vi "test.vi"() -> ()   [LabVIEW 2024]
uses:
  src/Zero Timeout Message Handler/~Message/~Message.lvclass
  PID Loop/PID Loop/PID Loop.lvclass
  PID Loop/PID Loop/Loop Msg/Loop Msg.lvclass
  C:/Users/uspoaotto/OneDrive - Oregon Tool/Desktop/working copies/zeroTimeoutMessageHandler/src/Zero Timeout Message Handler/~Message/~Message.lvclass
  src/Zero Timeout Message Handler/Start Polling Msg/Start Polling Msg.lvclass
  src/Zero Timeout Message Handler/Set Polling Message Msg/Set Polling Message Msg.lvclass
  src/Zero Timeout Message Handler/Stop Polling Msg/Stop Polling Msg.lvclass
  src/Zero Timeout Message Handler/Stop Msg/Stop Msg.lvclass
  PID Loop/PID Loop/Set Loop Period Msg/Set Loop Period Msg.lvclass
panel:
  in  "Loop Period (ms)":u32=10
  in  "stop polling":bool
  in  "start polling":bool
  in  "launch PID loop":bool
  in  "stop":bool
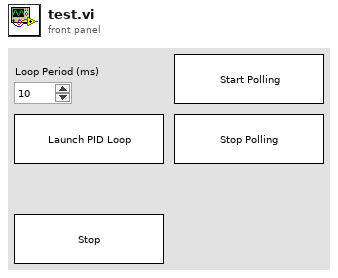
[diagram p1: front panel]
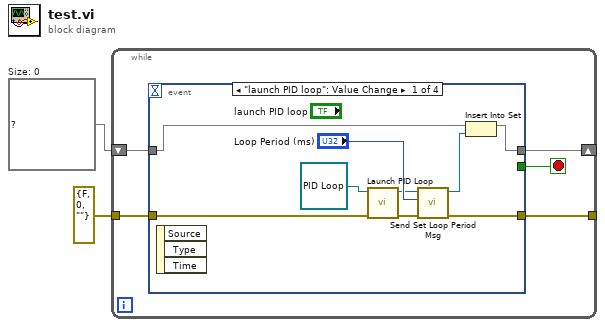
[diagram p0: block diagram]
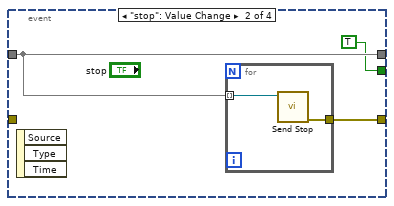
[diagram p2: hidden frame]
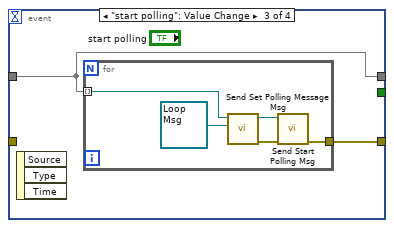
[diagram p3: hidden frame]
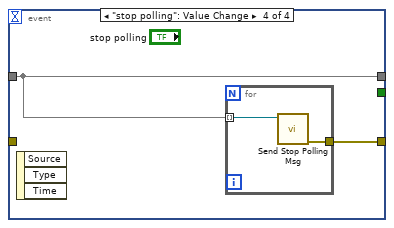
[diagram p4: hidden frame]
diagram:
  w2 = set{refnum<queue>} {}  # Size: 0
  n1 = while {
    shift-right: [w5] -> _
    shift-left: w2 -> [w4]
    tunnel: [w7] -> _
    tunnel: errorcluster {"status"=FALSE, "code"=0, "source"=""} ("error constant") -> [w3]
    stop <- w6 stop-if-true
    n2 = event shown="[0] \"launch PID loop\": Value Change" {
      selector: _ -> [_ _ _ _]
      dyn-events: _ -> [_ _ _ _]
      timeout: _ -> [_ _ _ _]
      tunnel: w4 -> [w16 w18 w23 w30]
      tunnel: [w15 w18 w23 w30] -> w5
      tunnel: [w10 w19 w22 w29] -> w7
      tunnel: [_ TRUE _ _] -> w6
      tunnel: w3 -> [w8 _ _ _]
      event "launch PID loop": Value Change {
        n3 = event-data() -> ()  [unwired: 1 in, 3 out]
        n4 = call "Launch PID Loop.vi"("error in (no error)"=w8, "PID Loop"=refnum<class "PID Loop.lvclass"> refnum ("PID Loop.lvlib:PID Loop.lvclass")) -> ("error out"=w9:errorcluster, "Message Queue out"=w12:refnum<queue>)  [unwired: 7 in, 1 out]
        n5 = call "Send Set Loop Period Msg.vi"("error in (no error)"=w9, "Loop Period in ms (10)"="Loop Period (ms)", "Message Queue in"=w12) -> ("error out"=w10:errorcluster, "Message Queue out"=w11:refnum<queue>)  [unwired: 7 in]
        n6 = Insert Into Set(10:w11, 11:w16) -> (3:w15:set{refnum<queue>})  [unwired: 1 out]
      }
      event "stop": Value Change {
        n7 = event-data() -> ()  [unwired: 1 in, 3 out]
        n8 = for {
          tunnel: w18 -> [w21] mode=indexing
          tunnel: [w20] -> w19
          n9 = call "Send Stop.vi"("Message Queue"=w21) -> ("error out"=w20:errorcluster)  [unwired: 10 in]
        }
      }
      event "start polling": Value Change {
        n10 = event-data() -> ()  [unwired: 1 in, 3 out]
        n11 = for {
          tunnel: w23 -> [w24] mode=indexing
          tunnel: [w25] -> w22
          n12 = call "Send Set Polling Message Msg.vi"("Polling Message"=refnum<class "Loop Msg.lvclass"> refnum ("PID Loop.lvlib:Loop Msg.lvclass"), "Message Queue in"=w24) -> ("error out"=w28:errorcluster, "Message Queue out"=w27:refnum<queue>)  [unwired: 8 in]
          n13 = call "Send Start Polling Msg.vi"("error in (no error)"=w28, "Message Queue in"=w27) -> ("error out"=w25:errorcluster)  [unwired: 8 in, 1 out]
        }
      }
      event "stop polling": Value Change {
        n14 = event-data() -> ()  [unwired: 1 in, 3 out]
        n15 = for {
          tunnel: w30 -> [w32] mode=indexing
          tunnel: [w31] -> w29
          n16 = call "Send Stop Polling Msg.vi"("Message Queue out"=w32) -> ("error out"=w31:errorcluster)  [unwired: 9 in, 1 out]
        }
      }
    }
  }
